vi "ziIDToServer.vi"(8 "Error In":errorcluster, 10 "Conn In":u64, 11 "Device ID":string="DEV209") -> (0 "Error Out":errorcluster, 2 "Conn Out":u64, 3 "ziDiscovery":T1={"timestamp"=0, "deviceid"="", "devicetype"="", "serveraddress"="", "serverport"=0, "apilevel"=0, "discoverable"=TRUE, "interface"="", "connected"="", "available"=TRUE, "owner"="", "status"="", "options "=""})   [LabVIEW 2016, in "Zurich Instruments LabOne.lvlib"]
doc: "Enter the Device ID, e.g., \"DEV2003\", to receive the standard input for ziOpen.vi."
uses:
  Zurich Instruments LabOne.lvlib
  ziTypeDisovery.ctl
  Private/ziLV64.framework
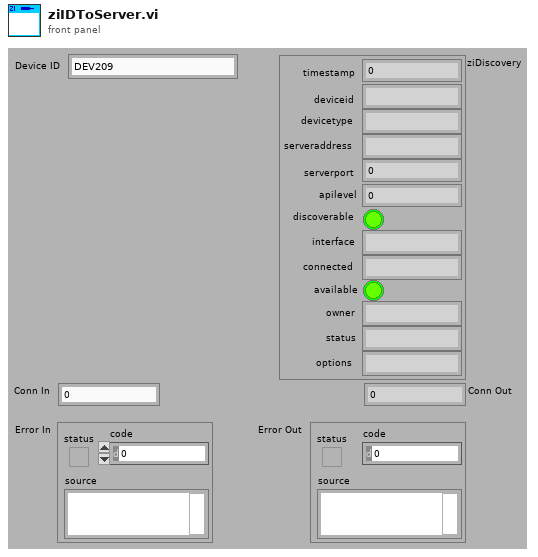
[diagram p1: front panel]
types:
  T1 = typedef "ziTypeDisovery.ctl" = cluster{"timestamp":u64, "deviceid":string, "devicetype":string, "serveraddress":string, "serverport":u32, "apilevel":u32, "discoverable":bool, "interface":string, "connected":string, "available":bool, "owner":string, "status":string, "options ":string}
  T2 = cluster{u64, u8[], u8[], u8[], u32, u32, bool, u8[], u8[], bool, u8[], u8[], u8[]}
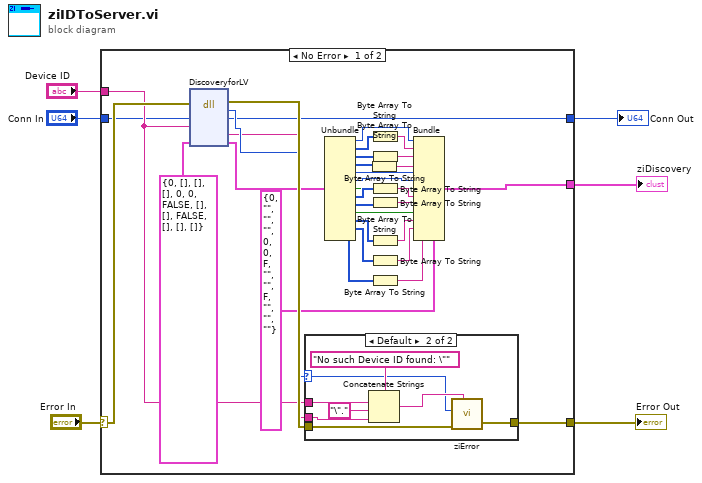
[diagram p0: block diagram]
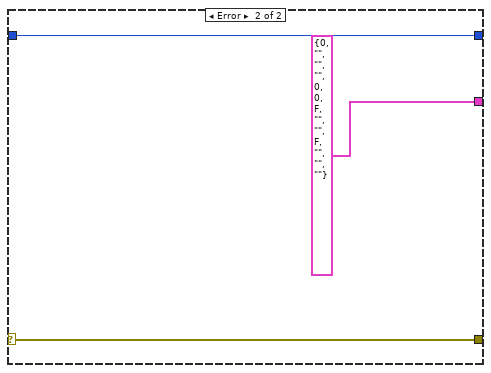
[diagram p3: hidden frame]
diagram:
  n1 = case shown="No Error" "Error In" {
    selector: "Error In" -> [w39 w51]
    tunnel: [w19 w51] -> w4
    tunnel: "Device ID" -> [w37 _]
    tunnel: [w30 T1 {"timestamp"=0, "deviceid"="", "devicetype"="", "serveraddress"="", "serverport"=0, "apilevel"=0, "discoverable"=FALSE, "interface"="", "connected"="", "available"=FALSE, "owner"="", "status"="", "options "=""} ("ziDiscoverHandle 2")] -> w3
    tunnel: "Conn In" -> [w21 w49]
    tunnel: [w20 w49] -> w1
    frame No Error {
      n2 = dll-call lib="Users/arkady/Desktop/ado/github/resonant_ultrasound_arxiv/maglab ultrasound -- arkady --arxiv/Zurich/Zurich Instruments/LabOne/API/LabVIEW/Zurich Instruments LabOne/Private/ziLV*.*" fn="DiscoveryforLV"(error in=w39, "conn"=w21, "deviceSerial"=w37, "DiscoveryObj"=T2 {0, [], [], [], 0, 0, FALSE, [], [], FALSE, [], [], []}) -> (error out=w38:errorcluster, "return type"=w36:u32, "conn"=w20:u64, "ErrorMsg"=w35:string, "DiscoveryObj"=w34:T2)  [unwired: 4 in, 1 out]
      n3 = case shown="Default" w36 {
        selector: w36 -> [_ w42]
        tunnel: w38 -> [w40 w48]
        tunnel: [w40 w47] -> w19
        tunnel: w37 -> [_ w43]
        tunnel: w35 -> [_ w41]
        frame 0 {
        }
        frame Default {
          n4 = Concatenate Strings("No such Device ID found: \"" ("source"), w43, "\"." ("source"), w41) -> (w44:string)
          n5 = call "ziError.vi"("ziErrorCode"=w42, "Error In"=w48, "Annotation"=w44) -> ("Error Out"=w47:errorcluster)  [unwired: 2 in, 1 out]
        }
      }
      n6 = Unbundle(w34) -> (w28:u64, w32:u8[], w31:u8[], w10:u8[], w11:u32, w12:u32, w13:bool, w15:u8[], w16:u8[], w14:bool, w25:u8[], w24:u8[], w8:u8[])
      n7 = Byte Array To String(unsigned byte array=w10) -> (string=w9:string)
      n8 = Byte Array To String(unsigned byte array=w32) -> (string=w26:string)
      n9 = Byte Array To String(unsigned byte array=w31) -> (string=w27:string)
      n10 = Byte Array To String(unsigned byte array=w15) -> (string=w17:string)
      n11 = Byte Array To String(unsigned byte array=w16) -> (string=w18:string)
      n12 = Byte Array To String(unsigned byte array=w25) -> (string=w22:string)
      n13 = Byte Array To String(unsigned byte array=w24) -> (string=w23:string)
      n14 = Byte Array To String(unsigned byte array=w8) -> (string=w7:string)
      n15 = Bundle(cluster=T1 {"timestamp"=0, "deviceid"="", "devicetype"="", "serveraddress"="", "serverport"=0, "apilevel"=0, "discoverable"=FALSE, "interface"="", "connected"="", "available"=FALSE, "owner"="", "status"="", "options "=""} ("ziDiscoverHandle 2"), "timestamp"=w28, "deviceid"=w26, "devicetype"=w27, "serveraddress"=w9, "serverport"=w11, "apilevel"=w12, "discoverable"=w13, "interface"=w17, "connected"=w18, "available"=w14, "owner"=w22, "status"=w23, "options"=w7) -> (w30:T1)
    }
    frame Error {
    }
  }
  "Error Out" <- w4
  "ziDiscovery" <- w3
  "Conn Out" <- w1
